vi "FilterComparison.vi"() -> ()   [LabVIEW 2019]
uses:
  <vilib>/Rock Robotics/WPI/ThirdParty/JAS_Junk/TrajLib/LinearFilter_ResetToValue.vi
  <vilib>/Rock Robotics/WPI/ThirdParty/JAS_Junk/TrajLib/LinearFilter_Calculate.vi
  <vilib>/Rock Robotics/WPI/ThirdParty/JAS_Junk/TrajLib/MedianFilter_New.vi
  <vilib>/Rock Robotics/WPI/ThirdParty/JAS_Junk/TrajLib/MedianFilter_ResetToValue.vi
  <vilib>/Rock Robotics/WPI/ThirdParty/JAS_Junk/TrajLib/MathUtil_Clamp.vi
  <vilib>/Rock Robotics/WPI/ThirdParty/JAS_Junk/TrajLib/MedianFilter_Calculate.vi
  <vilib>/Rock Robotics/WPI/ThirdParty/JAS_Junk/TrajLib/LinearFilter_MovingAverage.vi
  <vilib>/Rock Robotics/WPI/ThirdParty/JAS_Junk/TrajLib/LinearFilter_LowPassBW1.vi
  <vilib>/Rock Robotics/WPI/ThirdParty/JAS_Junk/TrajLib/LinearFilter_LowPassBW2.vi
  <vilib>/Rock Robotics/WPI/ThirdParty/JAS_Junk/TrajLib/LinearFilter_HighPassBW1.vi
  <vilib>/Rock Robotics/WPI/ThirdParty/JAS_Junk/TrajLib/LinearFilter_HighPassBW2.vi
  <vilib>/Rock Robotics/WPI/ThirdParty/JAS_Junk/TrajLib/Trajectory_Library.lvlib
panel:
  out "Wait Adjust":dbl format="%11.3f"
  in  "Auto / Manual":bool=TRUE
  in  "Enable\nNoise":bool=TRUE
  in  "Filter Enable":bool=TRUE
  in  "Use White Noise":bool=TRUE
  in  "Tab Control 2":T1(tab)
  out "Avg3":cluster{dbl, dbl, "Value_Output":dbl}(graph)
  out "Avg3 Out Dial":dbl(knob)=-2.895988890827539e-05 scale=-20.0..20.0
  out "Avg3 Out":dbl format="%11.3f"
  out "Med3":cluster{dbl, dbl, "Value_Output":dbl}(graph)
  out "Med3 Out":dbl format="%11.3f"
  out "Med3 Out Dial":dbl(knob)=-2.895988890827539e-05 scale=-20.0..20.0
  out "Avg7":cluster{dbl, dbl, "Value_Output":dbl}(graph)
  out "Avg7 Out":dbl format="%11.3f"
  out "Avg7 Out Dial":dbl(knob)=-2.895988890827539e-05 scale=-20.0..20.0
  out "Med7":cluster{dbl, dbl, "Value_Output":dbl}(graph)
  out "Med7 Out":dbl format="%11.3f"
  out "Med7 Out Dial":dbl(knob)=-2.895988890827539e-05 scale=-20.0..20.0
  out "LP BW 2":cluster{dbl, dbl, "Output_Value":dbl}(graph)
  out "LP BW 1 Out":dbl format="%11.3f"
  out "Low Pass 1st order Butterworth FIlter":dbl(knob)=-2.895988890827539e-05 scale=-20.0..20.0
  out "Fc 2":dbl format="%11.3f"
  out "LP BW 2":cluster{dbl, dbl, "Output_Value":dbl}(graph)
  out "LP BW 2 Out":dbl format="%11.3f"
  out "Low Pass 2nd order Butterworth Filter":dbl(knob)=-2.895988890827539e-05 scale=-20.0..20.0
  out "Fc 3":dbl format="%11.3f"
  out "HP BW 1":cluster{dbl, dbl, "Output_Value":dbl}(graph)
  out "HP BW 1":dbl format="%11.3f"
  out "High Pass 1st order Butterworth Filter":dbl(knob)=-2.895988890827539e-05 scale=-20.0..20.0
  out "HP  BW 2":cluster{dbl, dbl, "Output_Value":dbl}(graph)
  out "HP BW 2 out":dbl format="%11.3f"
  out "High Pass 2nd order Butterworth Filter":dbl(knob)=-2.895988890827539e-05 scale=-20.0..20.0
  out "Cutoff Freq\nHP BW 2":dbl format="%11.3f"
  out "Duration":dbl format="%11.3f"
  out "Late":dbl format="%11.3f"
  in  "Manual\nInput":dbl(slide) min=-12.0 max=12.0 scale=-12.0..12.0
  out "Raw Noise":dbl(knob)=-2.895988890827539e-05 scale=-20.0..20.0
  out "Raw Noise":dbl format="%11.3f"
  out "Actual Input":dbl(knob)=-2.895988890827539e-05 scale=-20.0..20.0
  out "Actual Input":dbl format="%11.3f"
  in  "Time Const (Sec)":dbl=0.08 min=0.0 step=0.001 format="%10.4f"
  out "Input":cluster{"Manual\nInput":dbl, dbl, "f":dbl}(graph)
  out "Meas Dial":dbl(knob)=-2.895988890827539e-05 scale=-20.0..20.0
  out "Measured Value":dbl format="%11.3f"
  # "Comparison of Different Filters"
  # "Loop Information"
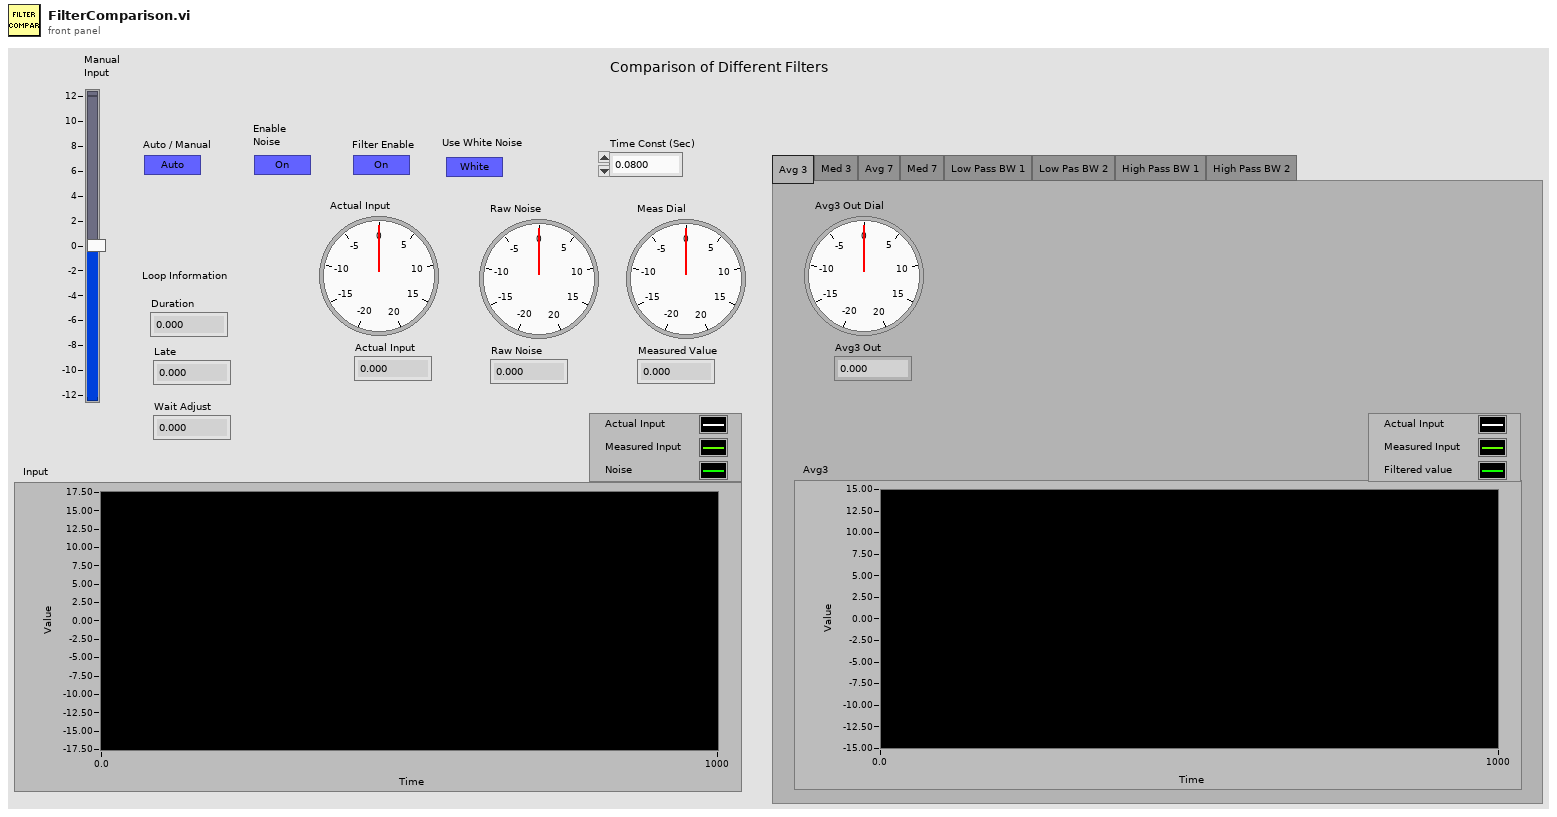
[diagram p1: front panel]
types:
  T1 = enum32{"Avg 3", "Med 3", "Avg 7", "Med 7", "Low Pass BW 1", "Low Pas BW 2", "High Pass BW 1", "High Pass BW 2"}
  T2 = enum16{"Moving Average", "Low Pass 1st Order Butterworth", "Low Pass 2nd Order Butterworth", "High Pass 1st Order Butterworth", "High Pass 2nd Order Butterworth"}
  T3 = cluster{"Manual\nInput":dbl, dbl, "MedianValue":dbl}
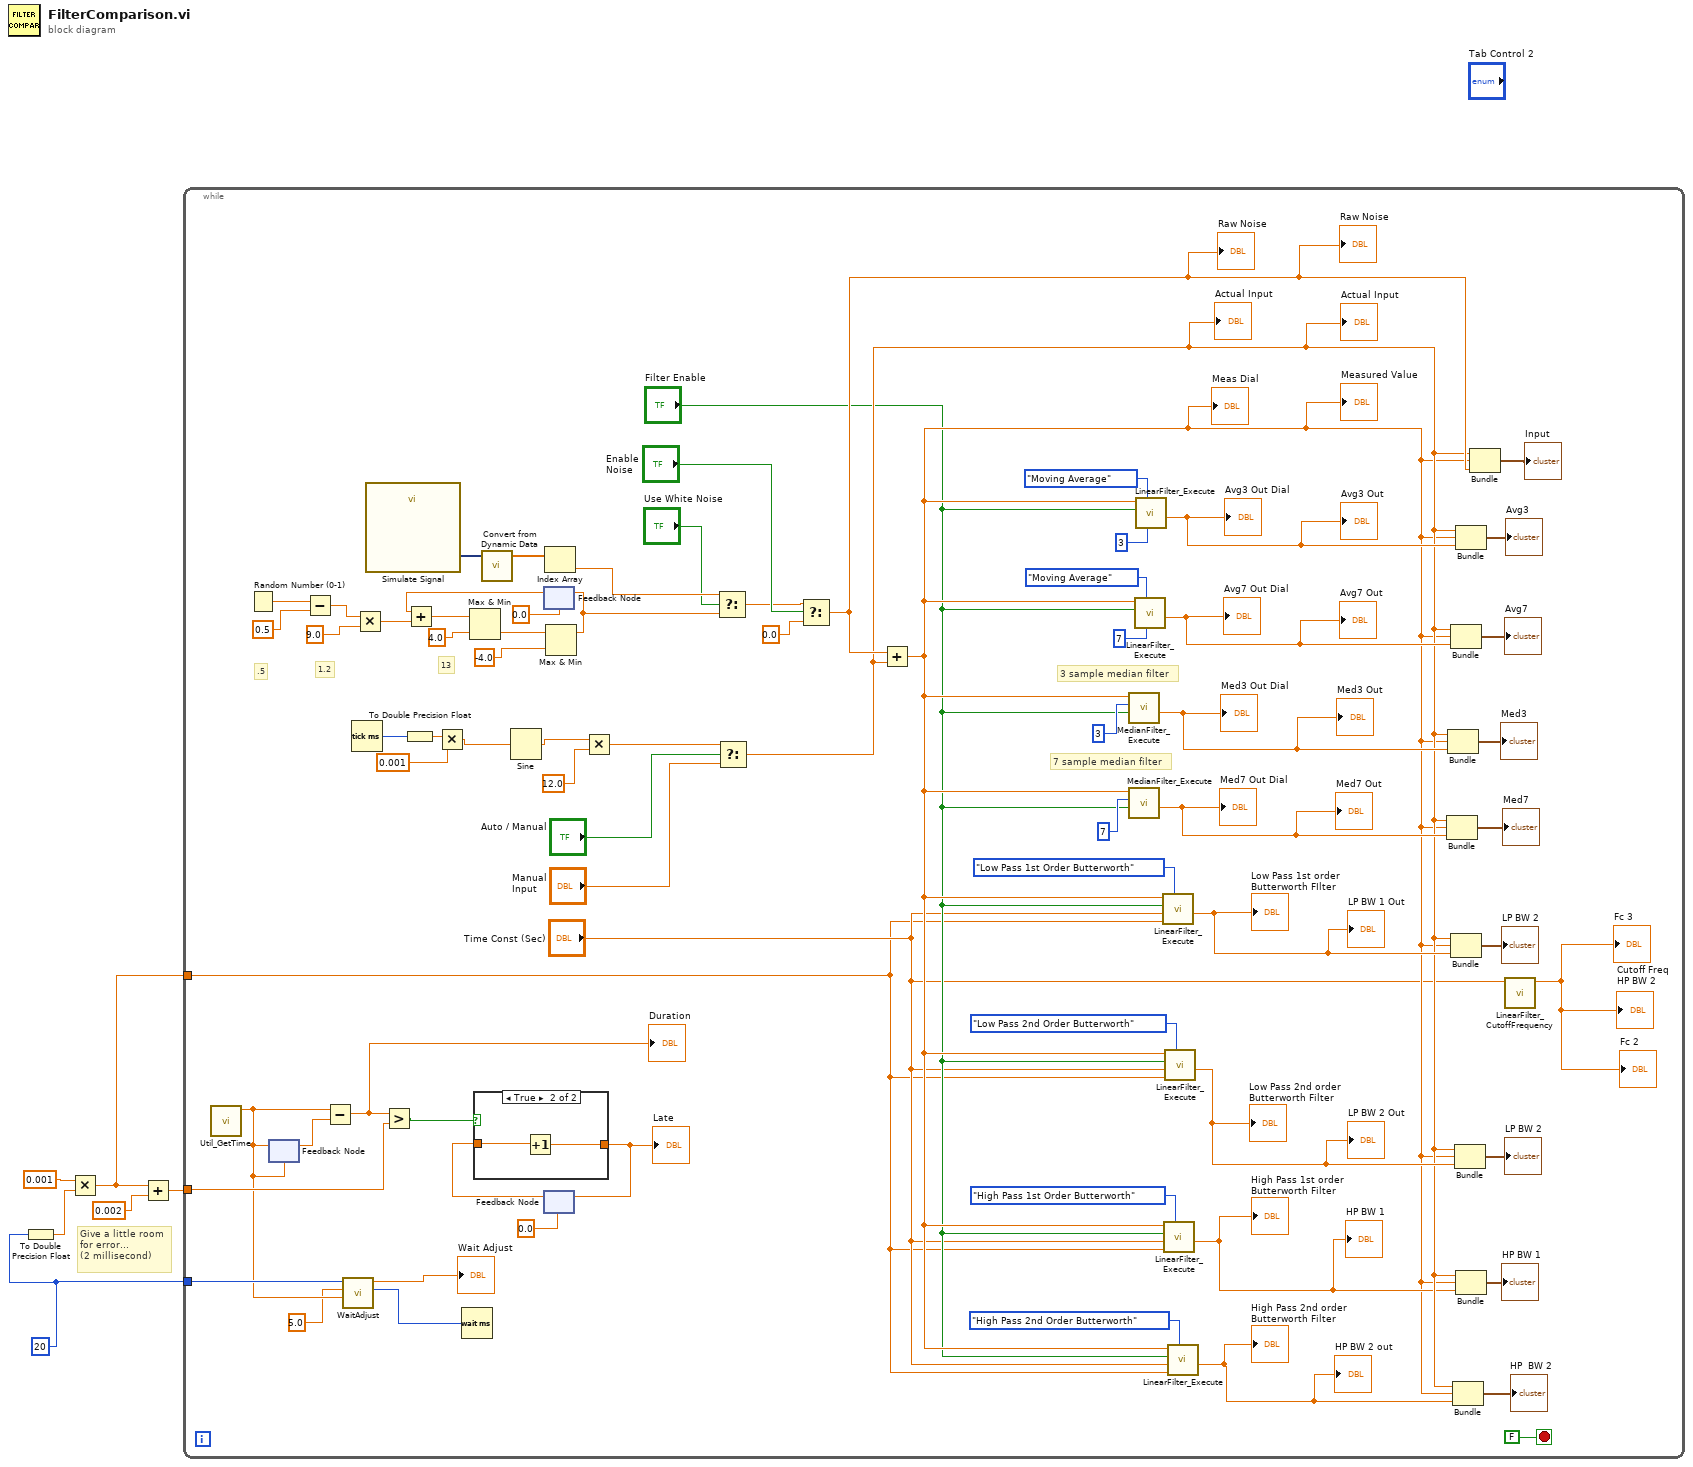
[diagram p0: block diagram]
diagram:
  w4 = u32 20 ("milliseconds to wait")
  # "Give a little room\nfor error...\n(2 millisecond)"
  n1 = To Double Precision Float(number=w4) -> (double precision float=w6:dbl)
  n2 = Multiply(x=0.001, y=w6) -> (x*y=w1:dbl)
  n3 = Add(x=w1, y=0.002) -> (x+y=w3:dbl)
  n4 = while {
    tunnel: w4 -> [w11]
    tunnel: w3 -> [w36]
    tunnel: w1 -> [w13]
    stop <- FALSE stop-if-true
    # "7 sample median filter"
    # "3 sample median filter"
    # "13"
    # "1.2"
    # ".5"
    n5 = call <vilib>:"Util_GetTime.vi"() -> ("FPGA_Time_Seconds"=w10:dbl)  [unwired: 10 in, 1 out]
    n6 = Random Number (0-1)() -> (number: 0 to 1=w76:dbl)
    n7 = feedback-in #1(w10) -> ()
    n8 = feedback #1(w10) -> (w39:dbl)
    n9 = Subtract(x=w76, y=0.5) -> (x-y=w72:dbl)
    n10 = Subtract(x=w10, y=w39) -> (x-y=w37:dbl)
    "Duration" <- w37
    n11 = call <vilib>:"WaitAdjust.vi"("Time_SEC"=w10, "MaxDeviation_MS"=5.0, "DesiredLoopTime_MS"=w11) -> ("AdjustedWaitTime_MS"=w8:u32, "Offset_MS"=→"Wait Adjust":dbl)  [unwired: 7 in]
    n12 = Tick Count (ms)() -> (millisecond timer value=w65:u32)
    n13 = Multiply(x=w72, y=9.0) -> (x*y=w71:dbl)
    n14 = call "Simulate Signal"() -> ("DC with Uniform Noise"=w53:dynamicdata)  [unwired: 14 in, 1 out]
    n15 = Greater?(x=w37, y=w36) -> (0:w38:bool)
    n16 = To Double Precision Float(number=w65) -> (double precision float=w66:dbl)
    n17 = Multiply(x=w66, y=0.001) -> (x*y=w63:dbl)
    n18 = Wait (ms)(milliseconds to wait=w8) -> ()  [unwired: 1 out]
    n19 = call "Convert from Dynamic Data"("Dynamic Data Type"=w53) -> ("Array"=w52:dbl[])  [unwired: 3 in]
    n20 = Sine(x=w63) -> (sin(x)=w62:dbl)
    n21 = feedback #2(0.0) -> (w73:dbl)
    n22 = Add(x=w73, y=w71) -> (x+y=w75:dbl)
    n23 = Max & Min(x=w75, y=4.0) -> (min(x,y)=w74:dbl)  [unwired: 1 out]
    n24 = feedback #3(0.0) -> (w46:dbl)
    n25 = case shown="True" w38 {
      tunnel: [w82 w84] -> w47
      tunnel: w46 -> [w82 w83]
      frame False {
      }
      frame True {
        n26 = Increment(x=w83) -> (x+1=w84:dbl)
      }
    }
    "Late" <- w47
    n27 = feedback-in #3(w47) -> ()
    n28 = Index Array(array=w52) -> (element=w51:dbl)  [unwired: 1 in]
    n29 = Max & Min(x=w74, y=-4.0) -> (max(x,y)=w54:dbl)  [unwired: 1 out]
    n30 = feedback-in #2(w54) -> ()
    n31 = Multiply(x=w62, y=12.0) -> (x*y=w59:dbl)
    n32 = Select(t=w51, s="Use White Noise", f=w54) -> (s? t:f=w55:dbl)
    n33 = Select(t=w59, s="Auto / Manual", f="Manual\nInput") -> (s? t:f=w21:dbl)
    "Actual Input" <- w21
    "Actual Input" <- w21
    n34 = Select(t=w55, s="Enable\nNoise", f=0.0) -> (s? t:f=w49:dbl)
    "Raw Noise" <- w49
    "Raw Noise" <- w49
    n35 = Add(x=w49, y=w21) -> (x+y=w16:dbl)
    "Measured Value" <- w16
    "Meas Dial" <- w16
    n36 = call <vilib>:"MedianFilter_Execute.vi"("Enable"="Filter Enable", "Samples"=3, "Input Value"=w16) -> ("MedianValue"=w32:dbl)  [unwired: 7 in, 1 out]
    "Med3 Out" <- w32
    "Med3 Out Dial" <- w32
    n37 = call <vilib>:"MedianFilter_Execute.vi"("Enable"="Filter Enable", "Samples"=7, "Input Value"=w16) -> ("MedianValue"=w34:dbl)  [unwired: 7 in, 1 out]
    "Med7 Out" <- w34
    "Med7 Out Dial" <- w34
    n38 = call <vilib>:"LinearFilter_Execute.vi"("Samples"=7, "Filter Type"=T2."Moving Average", "Enable"="Filter Enable", "Input"=w16) -> ("Output"=w41:dbl)  [unwired: 6 in, 1 out]
    "Avg7 Out" <- w41
    "Avg7 Out Dial" <- w41
    n39 = call <vilib>:"LinearFilter_Execute.vi"("Samples"=3, "Filter Type"=T2."Moving Average", "Enable"="Filter Enable", "Input"=w16) -> ("Output"=w42:dbl)  [unwired: 6 in, 1 out]
    "Avg3 Out" <- w42
    "Avg3 Out Dial" <- w42
    n40 = call <vilib>:"LinearFilter_Execute.vi"("Filter Type"=T2."Low Pass 1st Order Butterworth", "SamplePeriod"=w13, "TimeConstant"="Time Const (Sec)", "Enable"="Filter Enable", "Input"=w16) -> ("Output"=w35:dbl)  [unwired: 5 in, 1 out]
    "LP BW 1 Out" <- w35
    "Low Pass 1st order Butterworth FIlter" <- w35
    n41 = call <vilib>:"LinearFilter_Execute.vi"("Filter Type"=T2."High Pass 1st Order Butterworth", "SamplePeriod"=w13, "TimeConstant"="Time Const (Sec)", "Enable"="Filter Enable", "Input"=w16) -> ("Output"=w17:dbl)  [unwired: 5 in, 1 out]
    "High Pass 1st order Butterworth Filter" <- w17
    "HP BW 1" <- w17
    n42 = call <vilib>:"LinearFilter_Execute.vi"("Filter Type"=T2."Low Pass 2nd Order Butterworth", "SamplePeriod"=w13, "TimeConstant"="Time Const (Sec)", "Enable"="Filter Enable", "Input"=w16) -> ("Output"=w24:dbl)  [unwired: 5 in, 1 out]
    "LP BW 2 Out" <- w24
    "Low Pass 2nd order Butterworth Filter" <- w24
    n43 = call <vilib>:"LinearFilter_Execute.vi"("Filter Type"=T2."High Pass 2nd Order Butterworth", "SamplePeriod"=w13, "TimeConstant"="Time Const (Sec)", "Enable"="Filter Enable", "Input"=w16) -> ("Output"=w18:dbl)  [unwired: 5 in, 1 out]
    "HP BW 2 out" <- w18
    "High Pass 2nd order Butterworth Filter" <- w18
    n44 = Bundle("Manual\nInput"=w21, w16, "MedianValue"=w34) -> (→"Med7":T3)  [unwired: 1 in]
    n45 = Bundle("Manual\nInput"=w21, w16, "MedianValue"=w32) -> (→"Med3":T3)  [unwired: 1 in]
    n46 = Bundle("Manual\nInput"=w21, w16, "Output"=w41) -> (→"Avg7":cluster{"Manual\nInput":dbl, dbl, "Output":dbl})  [unwired: 1 in]
    n47 = Bundle("Manual\nInput"=w21, w16, "Output"=w35) -> (→"LP BW 2":cluster{"Manual\nInput":dbl, dbl, "Output":dbl})  [unwired: 1 in]
    n48 = Bundle("Manual\nInput"=w21, w16, "Output"=w18) -> (→"HP  BW 2":cluster{"Manual\nInput":dbl, dbl, "Output":dbl})  [unwired: 1 in]
    n49 = Bundle("Manual\nInput"=w21, w16, "Output"=w24) -> (→"LP BW 2":cluster{"Manual\nInput":dbl, dbl, "Output":dbl})  [unwired: 1 in]
    n50 = Bundle("Manual\nInput"=w21, w16, "Output"=w42) -> (→"Avg3":cluster{"Manual\nInput":dbl, dbl, "Output":dbl})  [unwired: 1 in]
    n51 = Bundle("Manual\nInput"=w21, w16, "Output"=w17) -> (→"HP BW 1":cluster{"Manual\nInput":dbl, dbl, "Output":dbl})  [unwired: 1 in]
    n52 = Bundle("Manual\nInput"=w21, w16, "f"=w49) -> (→"Input":cluster{"Manual\nInput":dbl, dbl, "f":dbl})  [unwired: 1 in]
    n53 = call <vilib>:"LinearFilter_CutoffFrequency.vi"("TimeConstant"="Time Const (Sec)") -> ("Cutoff Freq"=→"Cutoff Freq\nHP BW 2" →"Fc 2" →"Fc 3":dbl)  [unwired: 10 in]
  }
